vi "TrajGen.vi"(9 "AnkleTraj":dbl[][](array[numeric])) -> (0 "XY Graph":cluster{"X":dbl, "Y":dbl}[](graph), 1 "AnkleTraj":T1[](array[typedef]), 2 "ToeOffIdx":i32, 3 "TrajLength":i32)   [LabVIEW 2015, in "ForceField.lvclass"]
uses:
  ForceField.lvclass
  TypeDef/AnkleTrajPt.ctl
  <vilib>/Analysis/baseanly.llb/Real Dot Product.vi
  <vilib>/Analysis/NI_AALBase.lvlib
panel:
  out "Waveform Graph":dbl[][](graph)
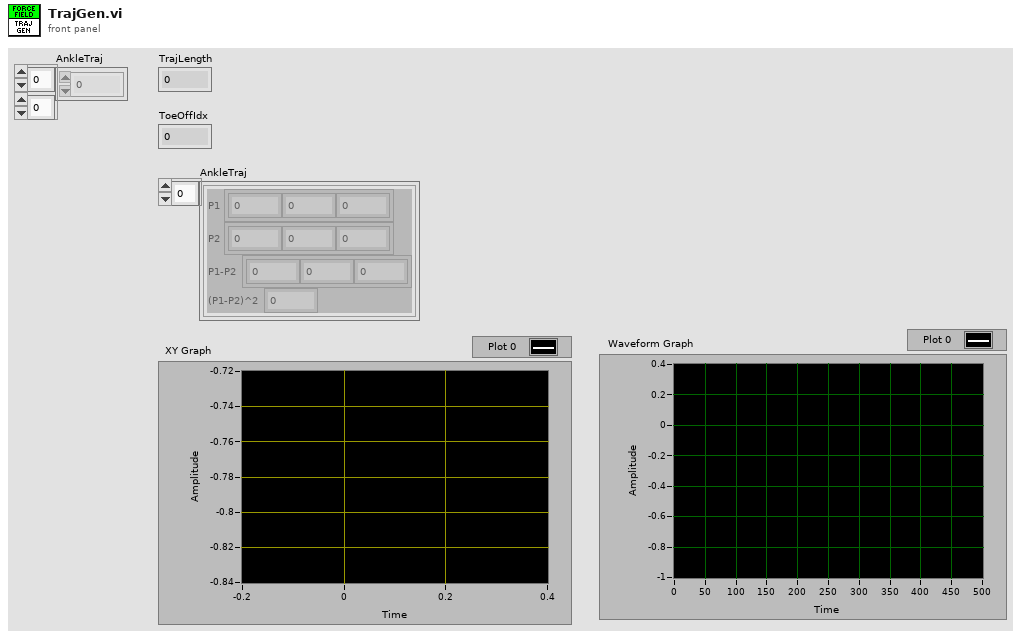
[diagram p1: front panel]
types:
  T1 = typedef "ForceField.lvclass/AnkleTrajPt.ctl" = cluster{"P1":dbl[], "P2":dbl[], "P1-P2":dbl[], "(P1-P2)^2":dbl}
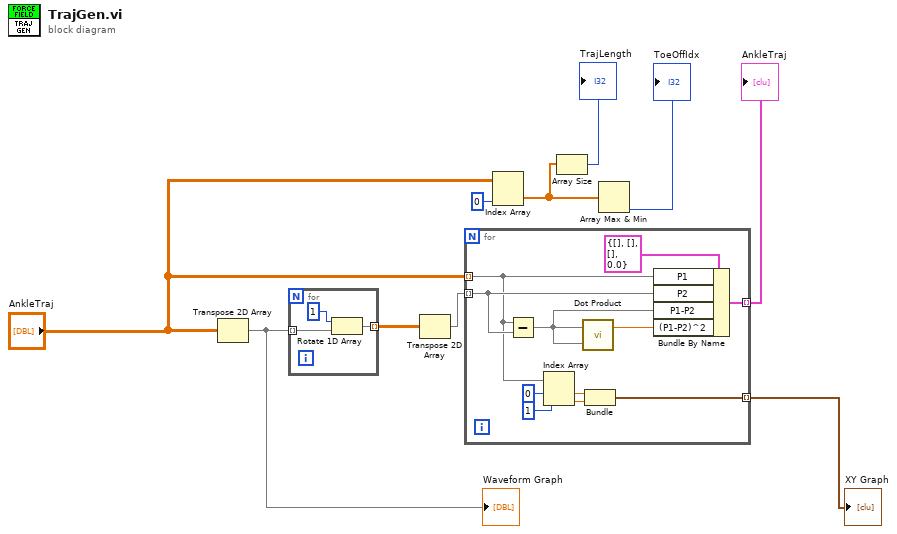
[diagram p0: block diagram]
diagram:
  n1 = Transpose 2D Array(2D array="AnkleTraj") -> (transposed array=w1:dbl[][])
  "Waveform Graph" <- w1
  n2 = for {
    tunnel: w1 -> [w13] mode=indexing
    tunnel: [w11] -> w4 mode=indexing
    n3 = Rotate 1D Array(1:w13, 2:1 ("n")) -> (0:w11:dbl[])
  }
  n4 = Transpose 2D Array(2D array=w4) -> (transposed array=w5:dbl[][])
  n5 = for {
    tunnel: "AnkleTraj" -> [w19] mode=indexing
    tunnel: [w24] -> w3 mode=indexing
    tunnel: w5 -> [w20] mode=indexing
    tunnel: [w16] -> w6 mode=indexing
    n6 = Subtract(x=w19, y=w20) -> (x-y=w22:dbl[])
    n7 = Index Array(array=w19, index #1=0 ("index"), index #2=1 ("index")) -> (element #1=w17:dbl, element #2=w18:dbl)
    n8 = call-poly <vilib>:"Dot Product.vi"("Y Vector"=w22, "X Vector"=w22) -> ("X * Y"=w21:dbl)  [unwired: 1 out]
    n9 = Bundle("element"=w17, "element"=w18) -> (w16:cluster{"element":dbl, "element":dbl})  [unwired: 1 in]
    n10 = Bundle By Name(cluster=T1 {"P1"=[], "P2"=[], "P1-P2"=[], "(P1-P2)^2"=0.0} ("AnkleTraj"), "P1"=w19, "P2"=w20, "P1-P2"=w22, "(P1-P2)^2"=w21) -> (w24:T1)
  }
  "XY Graph" <- w6
  "AnkleTraj" <- w3
  n11 = Index Array(array="AnkleTraj", index (col)=0 ("disabled index (col)")) -> (element=w9:dbl[])  [unwired: 1 in]
  n12 = Array Size(array=w9) -> (size(s)=→"TrajLength":i32)
  n13 = Array Max & Min(array=w9) -> (min index (indices)=→"ToeOffIdx":i32)  [unwired: 3 out]
